vi "SBML_Model_Info.vi"(8 "error in (no error)":errorcluster, 11 "Input SBML File":string) -> (0 "error out":errorcluster, 3 "Model Information":T1)   [LabVIEW 2014]
doc: "This VI extract the information of species' parameters present in SBML file. It takes the complete SBML file as input, and outputs: \nPr_Cnt --> How many parameters are there\nPr_Id_Arr --> Array of parameters\nPr_Name --> Array containing the name of parameters\nPr_Value --> Array containing the values of parameters\n\nDesigned by HB\nhaba@dtu.dk"
uses:
  Model Information.ctl
panel:
  out "Constant":string[](array[string])
  out "Units":string[](array[string])
  out "Pr_Value":string[](array[string])
  out "Pr_Name":string[](array[string])
  out "Pr_Id_Arr":string[](array[string])
  out "Model Info":string
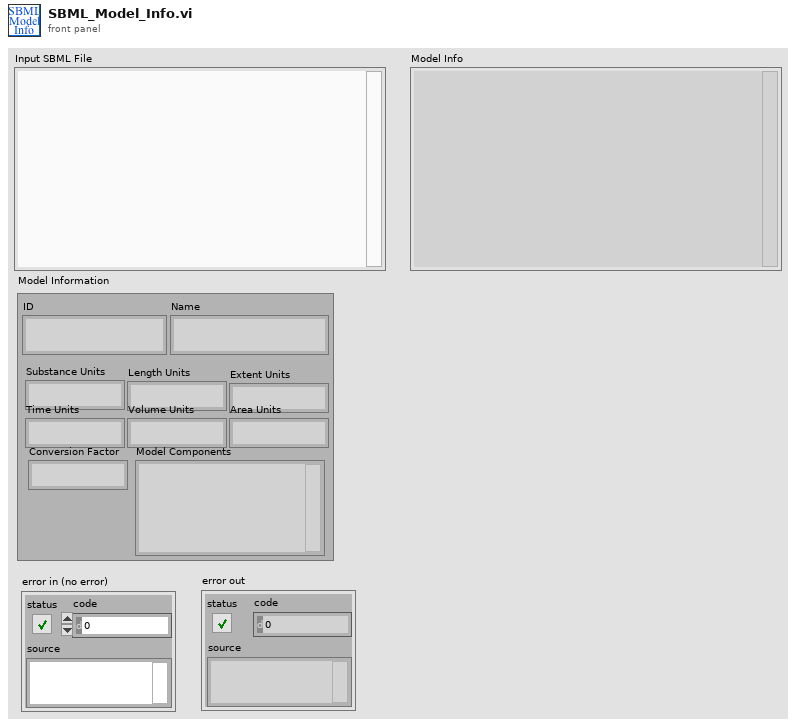
[diagram p1: front panel]
types:
  T1 = typedef "Model Information.ctl" = cluster{"ID":string, "Name":string, "Substance Units":string, "Time Units":string, "Volume Units":string, "Area Units":string, "Length Units":string, "Extent Units":string, "Conversion Factor":string, "Model Components":string}
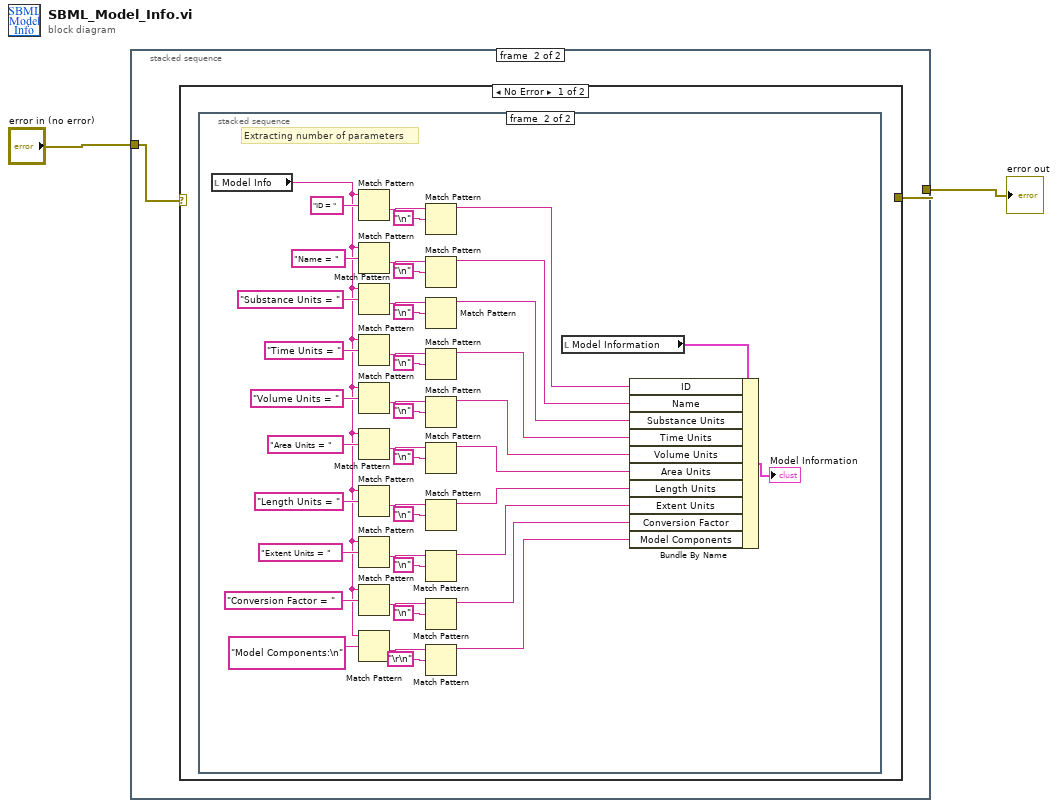
[diagram p0: block diagram]
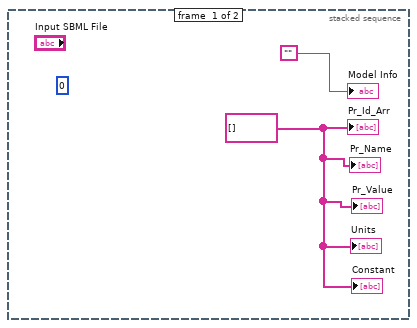
[diagram p2: hidden frame]
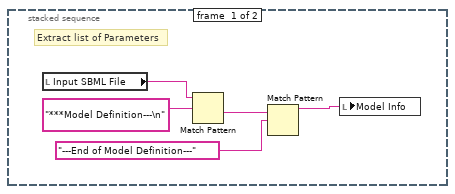
[diagram p3: hidden frame]
diagram:
  n1 = stacked-sequence {
    tunnel: "error in (no error)" -> [_ w5]
    tunnel: [_ w6] -> w1
    frame #0 {
      (unwired) 0 ("Sp_cnt")
      w3 = string[] [] ("Sp_Id_Arr")
      "Model Info" <- "" ("Full SBML File")
      "Pr_Id_Arr" <- w3
      "Pr_Name" <- w3
      "Pr_Value" <- w3
      "Units" <- w3
      "Constant" <- w3
    }
    frame #1 {
      n2 = case shown="No Error" w5 {
        selector: w5 -> [_ w55]
        tunnel: [_ w55] -> w6
        frame No Error {
          n3 = stacked-sequence {
            frame #0 {
              # "Extract list of Parameters"
              n4 = local read "Input SBML File"() -> (w10:string)
              n5 = Match Pattern(string=w10, regular expression="***Model Definition---\n") -> (after substring=w8:string)  [unwired: 1 in, 3 out]
              n6 = Match Pattern(string=w8, regular expression="---End of Model Definition---") -> (before substring=w11:string)  [unwired: 1 in, 3 out]
              n7 = local write "Model Info"(w11) -> ()
            }
            frame #1 {
              # "Extracting number of parameters"
              n8 = local read "Model Info"() -> (w24:string)
              n9 = Match Pattern(string=w24, regular expression="ID = ") -> (after substring=w52:string)  [unwired: 1 in, 3 out]
              n10 = Match Pattern(string=w24, regular expression="Name = ") -> (after substring=w51:string)  [unwired: 1 in, 3 out]
              n11 = Match Pattern(string=w24, regular expression="Substance Units = ") -> (after substring=w47:string)  [unwired: 1 in, 3 out]
              n12 = Match Pattern(string=w24, regular expression="Time Units = ") -> (after substring=w45:string)  [unwired: 1 in, 3 out]
              n13 = Match Pattern(string=w24, regular expression="Volume Units = ") -> (after substring=w40:string)  [unwired: 1 in, 3 out]
              n14 = Match Pattern(string=w24, regular expression="Area Units = ") -> (after substring=w39:string)  [unwired: 1 in, 3 out]
              n15 = Match Pattern(string=w24, regular expression="Length Units = ") -> (after substring=w27:string)  [unwired: 1 in, 3 out]
              n16 = Match Pattern(string=w24, regular expression="Extent Units = ") -> (after substring=w28:string)  [unwired: 1 in, 3 out]
              n17 = Match Pattern(string=w24, regular expression="Conversion Factor = ") -> (after substring=w33:string)  [unwired: 1 in, 3 out]
              n18 = Match Pattern(string=w24, regular expression="Model Components:\n") -> (after substring=w34:string)  [unwired: 1 in, 3 out]
              n19 = Match Pattern(string=w52, regular expression="\n") -> (before substring=w21:string)  [unwired: 1 in, 3 out]
              n20 = Match Pattern(string=w51, regular expression="\n") -> (before substring=w20:string)  [unwired: 1 in, 3 out]
              n21 = Match Pattern(string=w47, regular expression="\n") -> (before substring=w19:string)  [unwired: 1 in, 3 out]
              n22 = Match Pattern(string=w45, regular expression="\n") -> (before substring=w18:string)  [unwired: 1 in, 3 out]
              n23 = Match Pattern(string=w40, regular expression="\n") -> (before substring=w17:string)  [unwired: 1 in, 3 out]
              n24 = Match Pattern(string=w39, regular expression="\n") -> (before substring=w16:string)  [unwired: 1 in, 3 out]
              n25 = Match Pattern(string=w27, regular expression="\n") -> (before substring=w15:string)  [unwired: 1 in, 3 out]
              n26 = Match Pattern(string=w28, regular expression="\n") -> (before substring=w14:string)  [unwired: 1 in, 3 out]
              n27 = Match Pattern(string=w33, regular expression="\n") -> (before substring=w13:string)  [unwired: 1 in, 3 out]
              n28 = Match Pattern(string=w34, regular expression="\r\n") -> (before substring=w12:string)  [unwired: 1 in, 3 out]
              n29 = local read "Model Information"() -> (w22:T1)
              n30 = Bundle By Name(cluster=w22, "ID"=w21, "Name"=w20, "Substance Units"=w19, "Time Units"=w18, "Volume Units"=w17, "Area Units"=w16, "Length Units"=w15, "Extent Units"=w14, "Conversion Factor"=w13, "Model Components"=w12) -> (→"Model Information":T1)
            }
          }
        }
        frame Error {
        }
      }
    }
  }
  "error out" <- w1
